vi "Start_Client.vi"   [LabVIEW 2020]
types:
  T1 = cluster{"设备名称":string, "操作人员":string, "设备状态":enum16{"设备离线", "设备正常", "设备缺料", "设备故障", "质量报警"}, "附加信息":string}
  T2 = enum32{"Invalid", "Standard", "Closed", "Hidden", "Minimized", "Maximized"}
  T3 = cluster{"操作员编号":string, "操作员姓名":string, "操作员权限":string, "联机模式":enum16{"单机", "追溯"}}
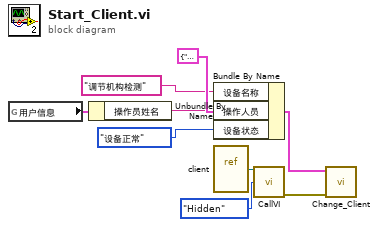
[diagram p0: block diagram]
diagram:
  n1 = global read "用户信息.vi" "用户信息"() -> (w3:T3)
  n2 = Unbundle By Name(w3) -> ("操作员姓名"=w2:string)
  n3 = Bundle By Name(cluster=T1 {"设备名称"="", "操作人员"="", "设备状态"=enum."设备离线", "附加信息"=""} ("设备信息"), "设备名称"="调节机构检测", "操作人员"=w2, "设备状态"=enum16{"设备离线", "设备正常", "设备缺料", "设备故障", "质量报警"}."设备正常") -> (w1:T1)
  n4 = vi-ref "client.vi"() -> (w9:refnum<vi>)
  n5 = call "CallVI.vi"("VI引用"=w9, "状态"=T2."Hidden") -> ("错误输出"=w7:errorcluster)  [unwired: 12 in, 1 out]
  n6 = call "Change_Client.vi"("错误输入（无错误）"=w7, "设备信息"=w1) -> ()  [unwired: 9 in, 1 out]
